vi "Example.vi"() -> ()   [LabVIEW 2014]
uses:
  <vilib>/Analysis/3filter.llb/FIR Filter (DBL).vi
  FrontPanelPublisher.lvlib
  <vilib>/Analysis/NI_AALBase.lvlib
  FrontPanelManager_class/FrontPanelManager.lvclass
panel:
  out "Progress":dbl(slide)=3.1645569620253164 scale=0.0..10.0
  in  "Path":path
  in  "Averaging":enum16{"5pt", "11pt", "33pt"}(ring)
  out "String":string
  out "<5":bool
  in  "Button":bool
  in  "Stop":bool
  out "XY Graph":cluster{i32[], "Filtered X":dbl[]}[](graph)
  in  "Append":bool
  in  "Numeric":dbl
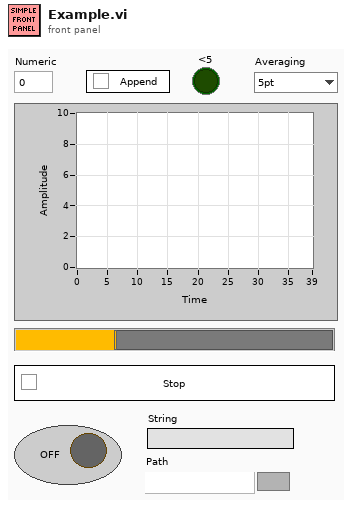
[diagram p1: front panel]
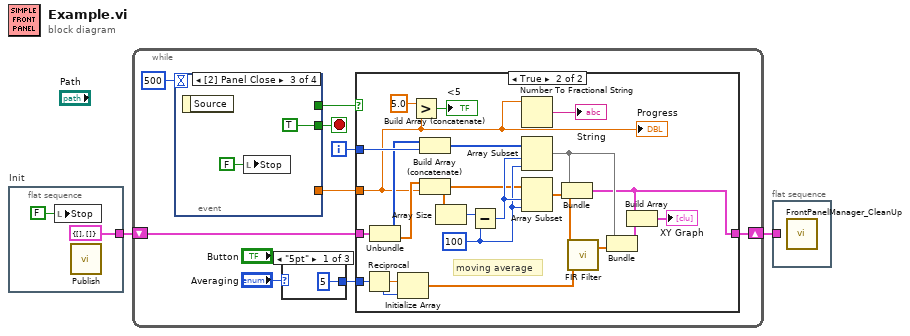
[diagram p0: block diagram]
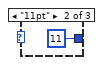
[diagram p2: hidden frame]
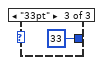
[diagram p3: hidden frame]
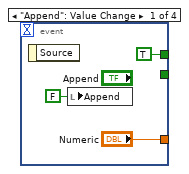
[diagram p5: hidden frame]
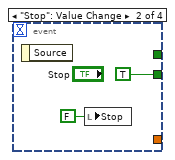
[diagram p6: hidden frame]
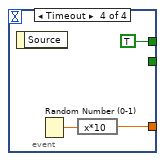
[diagram p7: hidden frame]
diagram:
  n1 = flat-sequence "Init" {
    tunnel: [cluster{i32[], dbl[]} {[], []} ("XY Graph")] -> w2
    frame #0 {
      n2 = local write "Stop"(FALSE ("Stop")) -> ()
      n3 = call "Publish.vi"() -> ()  [unwired: 12 in]
    }
  }
  n4 = while {
    shift-right: [w8] -> w1
    shift-left: w2 -> [w7]
    i -> [w10]
    stop <- w13 stop-if-true
    n5 = event shown="[2] Panel Close" {
      selector: _ -> [_ _ _ _]
      dyn-events: _ -> [_ _ _ _]
      timeout: 500 -> [_ _ _ _]
      tunnel: [_ TRUE TRUE _] -> w13
      tunnel: ["Numeric" _ _ w48] -> w9
      tunnel: [TRUE _ _ TRUE] -> w11
      event "Append": Value Change {
        n6 = event-data() -> ()  [unwired: 1 in, 1 out]
        n7 = local write "Append"(FALSE ("Add")) -> ()
      }
      event "Stop": Value Change {
        n8 = event-data() -> ()  [unwired: 1 in, 1 out]
        n9 = local write "Stop"(FALSE ("Stop")) -> ()
      }
      event Panel Close {
        n10 = event-data() -> ()  [unwired: 1 in, 1 out]
        n11 = local write "Stop"(FALSE ("Stop")) -> ()
      }
      event Timeout {
        n12 = event-data() -> ()  [unwired: 1 in, 1 out]
        n13 = Random Number (0-1)() -> (number: 0 to 1=w49:dbl)
        n14 = expression code="x*10"(w49) -> (w48:dbl)
      }
    }
    n15 = case shown="\"5pt\"" "Averaging" {
      tunnel: [5 11 33] -> w6
      frame "5pt" {
      }
      frame "11pt" {
      }
      frame "33pt" {
      }
    }
    n16 = case shown="True" w11 {
      tunnel: w10 -> [_ w39]
      tunnel: w9 -> [_ w18]
      tunnel: [w17 w24] -> w8
      tunnel: w7 -> [w17 w38]
      tunnel: w6 -> [_ w19]
      frame False {
      }
      frame True {
        w33 = 100 ("length")
        # "moving average"
        n17 = Reciprocal(x=w19) -> (1/x=w21:dbl)
        n18 = Unbundle(w38) -> (w36:i32[], w32:dbl[])
        n19 = Initialize Array(w21, w19) -> (w20:dbl[])
        n20 = Greater?(x=5.0, y=w18) -> (0:→"<5":bool)
        n21 = Build Array (concatenate)(w36, w39) -> (w37:i32[])
        n22 = Build Array (concatenate)(w32, w18) -> (w31:dbl[])
        n23 = Array Size(array=w31) -> (size(s)=w35:i32)
        n24 = Subtract(x=w35, y=w33) -> (x-y=w34:i32)
        n25 = Number To Fractional String(number=w18) -> (F-format string=→"String":string)  [unwired: 3 in]
        n26 = Array Subset(array=w37, index=w34, length=w33) -> (w27:i32[])
        n27 = Array Subset(array=w31, index=w34, length=w33) -> (w23:dbl[])
        n28 = Bundle(w27, w23) -> (w24:cluster{i32[], dbl[]})  [unwired: 1 in]
        n29 = call-poly <vilib>:"FIR Filter.vi"("FIR Coefficients"=w20, "X"=w23) -> ("Filtered X"=w22:dbl[])  [unwired: 2 in, 1 out]
        n30 = Bundle(w27, "Filtered X"=w22) -> (w25:cluster{i32[], "Filtered X":dbl[]})  [unwired: 1 in]
        n31 = Build Array(w24, w25) -> (→"XY Graph":cluster{i32[], "Filtered X":dbl[]}[])
        "Progress" <- w18
      }
    }
  }
  n32 = flat-sequence {
    tunnel: w1 -> [_]
    frame #0 {
      n33 = call "FrontPanelManager_CleanUp.vi"() -> ()  [unwired: 19 in, 1 out]
    }
  }
